vi "www template read file core.vi"(8 "error in (no error)":errorcluster, 11 "Path":path) -> (0 "error out":errorcluster, 2 "File Modified":timestamp, 3 "File Content":string)   [LabVIEW 2011]
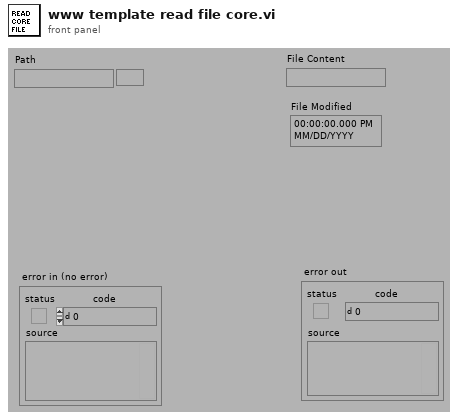
[diagram p1: front panel]
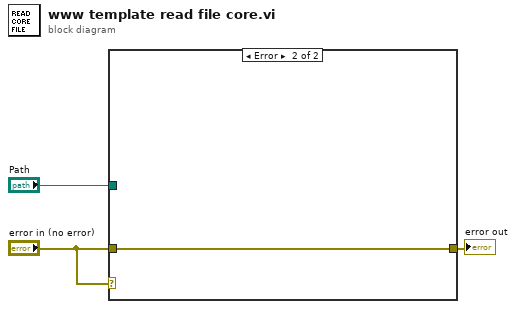
[diagram p0: block diagram]
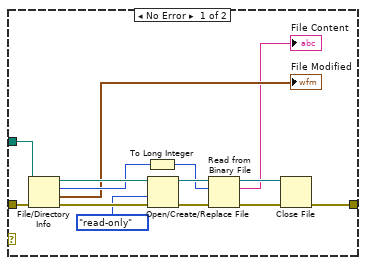
[diagram p2: hidden frame]
diagram:
  n1 = case shown="Error" "error in (no error)" {
    tunnel: [w6 w18] -> w3
    tunnel: "error in (no error)" -> [w5 w18]
    tunnel: "Path" -> [w4 _]
    frame No Error {
      n2 = File/Directory Info(path=w4, error in=w5) -> (path out=w11:path, size=w10:i64, last mod=→"File Modified":timestamp, error out=w17:errorcluster)  [unwired: 3 out]
      n3 = To Long Integer(number=w10) -> (32bit integer=w14:i32)
      n4 = Open/Create/Replace File(file path (use dialog)=w11, error in=w17, access (0:read/write)=enum16{"read/write", "read-only", "write-only"}."read-only") -> (refnum out=w15:refnum<file>, error out=w16:errorcluster)  [unwired: 4 out]
      n5 = Read from Binary File(8:w16, 10:w14, 11:w15) -> (0:w12:errorcluster, 2:→"File Content":string, 3:w13:refnum<file>)  [unwired: 4 out]
      n6 = Close File(refnum=w13, error in=w12) -> (error out=w6:errorcluster)  [unwired: 1 out]
    }
    frame Error {
    }
  }
  "error out" <- w3
